vi "Tolerance to Color Converter.vi"(2 "To select":T1=enum."Gold - 5%" caption="Tolerance select") -> (6 "Tol Color":u32(colorbox) caption="Tolerance Color")   [LabVIEW 2018, in "Enum to Color Converters.lvlib"]
doc: "Converts the selected Tolerance Enum value into the corresponding color for the resistor band."
uses:
  Enum to Color Converters.lvlib
  Tolerance--enum.ctl
  Resistor Band Colors/Resistor Band Colors.lvlib
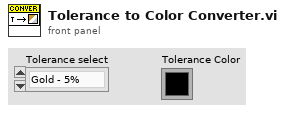
[diagram p1: front panel]
types:
  T1 = typedef "Tolerance--enum.ctl" = enum16{"Gray - 0.05%", "Violet - 0.1%", "Blue - 0.25%", "Green - 0.5%", "Brown - 1%", "Red - 2%", "Gold - 5%", "Silver - 10%", "None - 20%"}
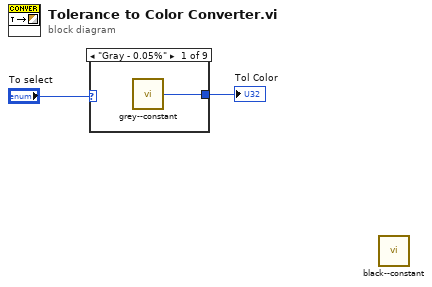
[diagram p0: block diagram]
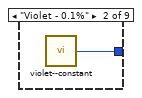
[diagram p2: hidden frame]
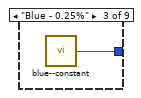
[diagram p3: hidden frame]
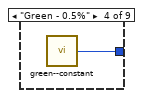
[diagram p4: hidden frame]
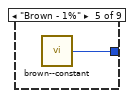
[diagram p5: hidden frame]
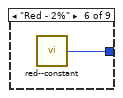
[diagram p6: hidden frame]
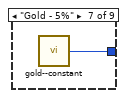
[diagram p7: hidden frame]
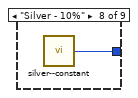
[diagram p8: hidden frame]
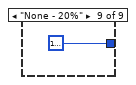
[diagram p9: hidden frame]
diagram:
  n1 = case shown="\"Gray - 0.05%\"" "To select" {
    tunnel: [w3 w4 w5 w6 w7 w8 w9 w10 u32 16777216] -> w1
    frame "Gray - 0.05%" {
      n2 = call "grey--constant.vi"() -> ("Gray"=w3:u32)  [unwired: 5 in]
    }
    frame "Violet - 0.1%" {
      n3 = call "violet--constant.vi"() -> ("Violet"=w4:u32)  [unwired: 5 in]
    }
    frame "Blue - 0.25%" {
      n4 = call "blue--constant.vi"() -> ("Blue"=w5:u32)  [unwired: 5 in]
    }
    frame "Green - 0.5%" {
      n5 = call "green--constant.vi"() -> ("Green"=w6:u32)  [unwired: 5 in]
    }
    frame "Brown - 1%" {
      n6 = call "brown--constant.vi"() -> ("Brown"=w7:u32)  [unwired: 5 in]
    }
    frame "Red - 2%" {
      n7 = call "red--constant.vi"() -> ("Red"=w8:u32)  [unwired: 5 in]
    }
    frame "Gold - 5%" {
      n8 = call "gold--constant.vi"() -> ("Gold"=w9:u32)  [unwired: 5 in]
    }
    frame "Silver - 10%" {
      n9 = call "silver--constant.vi"() -> ("Silver"=w10:u32)  [unwired: 5 in]
    }
    frame "None - 20%" {
    }
  }
  "Tol Color" <- w1
  n10 = call "black--constant.vi"() -> ()  [unwired: 5 in, 1 out]
